vi "Launcher.vi"() -> ()   [LabVIEW 2020]
uses:
  <vilib>/Analysis/6fits.llb/Curve Fitting Criteria.ctl
  <vilib>/Analysis/baseanly.llb/Mean (DBL).vi
  DAQ.lvlibp/D/BingoGithub/DAQ_V000.04/DAQ_Module/DAQ_Base_class/DAQ_Base.lvclass
  DAQ_Base_class/subvi/GlobalData_operation.ctl
  <vilib>/Analysis/NI_AALPro.lvlib
  <vilib>/Analysis/NI_AALBase.lvlib
panel:
  out "模拟量数量":i32
  out "自动采集第1段":dbl[][](graph)
  in  "Tab Control":enum32{"采集模块配置", "采集与调试", "模拟量标定"}(tab)
  in  "DAQSettings":T2={"SampleSettings"={"samples per channel"=100, "SampleRate"=1000.0, "TansMaxLength"=500000.0, "ReadTimeOut"=10.0, "时钟源"=""}, "AI_ChannelSettings"={"AI_SettingsArry"=[]}, "AO_ChannelSettings"={"布尔"=FALSE}, "Cnt_ChannelSettings"={"Cnt_ChannelSettings"=[]}} {"Cnt_ChannelSettings"."Cnt_ChannelSettings"."decoding type" items=["X1"=10090, "X2"=10091, "X4"=10092, "双脉冲计数"=10313]; "Cnt_ChannelSettings"."Cnt_ChannelSettings"."z index phase" items=["A High B High"=10040, "A High B Low"=10041, "A Low B High"=10042, "A Low B Low"=10043, ""=0]; "Cnt_ChannelSettings"."Cnt_ChannelSettings"."单位" items=["Radians"=10273, "Degrees"=10146, "Meters"=10219, "Inches"=10379, "Ticks"=10304, "From Custom Scale"=10065]; "AI_ChannelSettings"."AI_SettingsArry"."标定系数"."Offset" format="%_4g"; "AI_ChannelSettings"."AI_SettingsArry"."标定系数"."Scale" format="%.4g"; "AI_ChannelSettings"."AI_SettingsArry"."shunt resistor location" items=["默认"=-1, "内部"=10200, "外部"=10167]; "AI_ChannelSettings"."AI_SettingsArry"."external shunt resistor value" format="%0.2f"; "AI_ChannelSettings"."AI_SettingsArry"."输入信号类型" items=["默认"=-1, "RSE"=10083, "NRSE"=10078, "差分"=10106, "伪差分"=12529]; "AI_ChannelSettings"."AI_SettingsArry"."单位" items=["安培"=10342, "伏特"=10348, "来自自定义换算"=10065]}
  in  "Save":bool
  in  "ClearCurve":bool
  in  "数据采集通道使能":bool[](array[boolean])
  out "手动采集曲线":dbl[][](graph)
  in  "待标数据源":u16(ring) items=["输入轴扭矩", "输出轴扭矩"]
  in  "tb_sensor_calibrt_data":string[][](table) caption="标定点录入表"
  out "物理值曲线":dbl[](graph)
  in  "Play":bool
  in  "Add":bool
  in  "Remove":bool
  in  "Delete":bool
  in  "Calculate":bool
  in  "Download":bool
  out "real_value":dbl caption="实时值" format="%0.2f"
  out "mean":dbl caption="物理均值" format="%0.2f"
  out "标定拟合曲线":cluster{dbl[], "Best Linear Fit":dbl[]}[](graph)
  out "b_before":dbl caption="计算前偏移量"
  out "K_before":dbl caption="计算前线性度"
  in  "cal_K":dbl caption="计算后线性度"
  in  "cal_b":dbl caption="计算后偏移量"
  out "Stop":bool
  out "自动采集第2段":dbl[][](graph)
  in  "停止":bool
  out "RealTimeValue":dbl[](array[numeric])
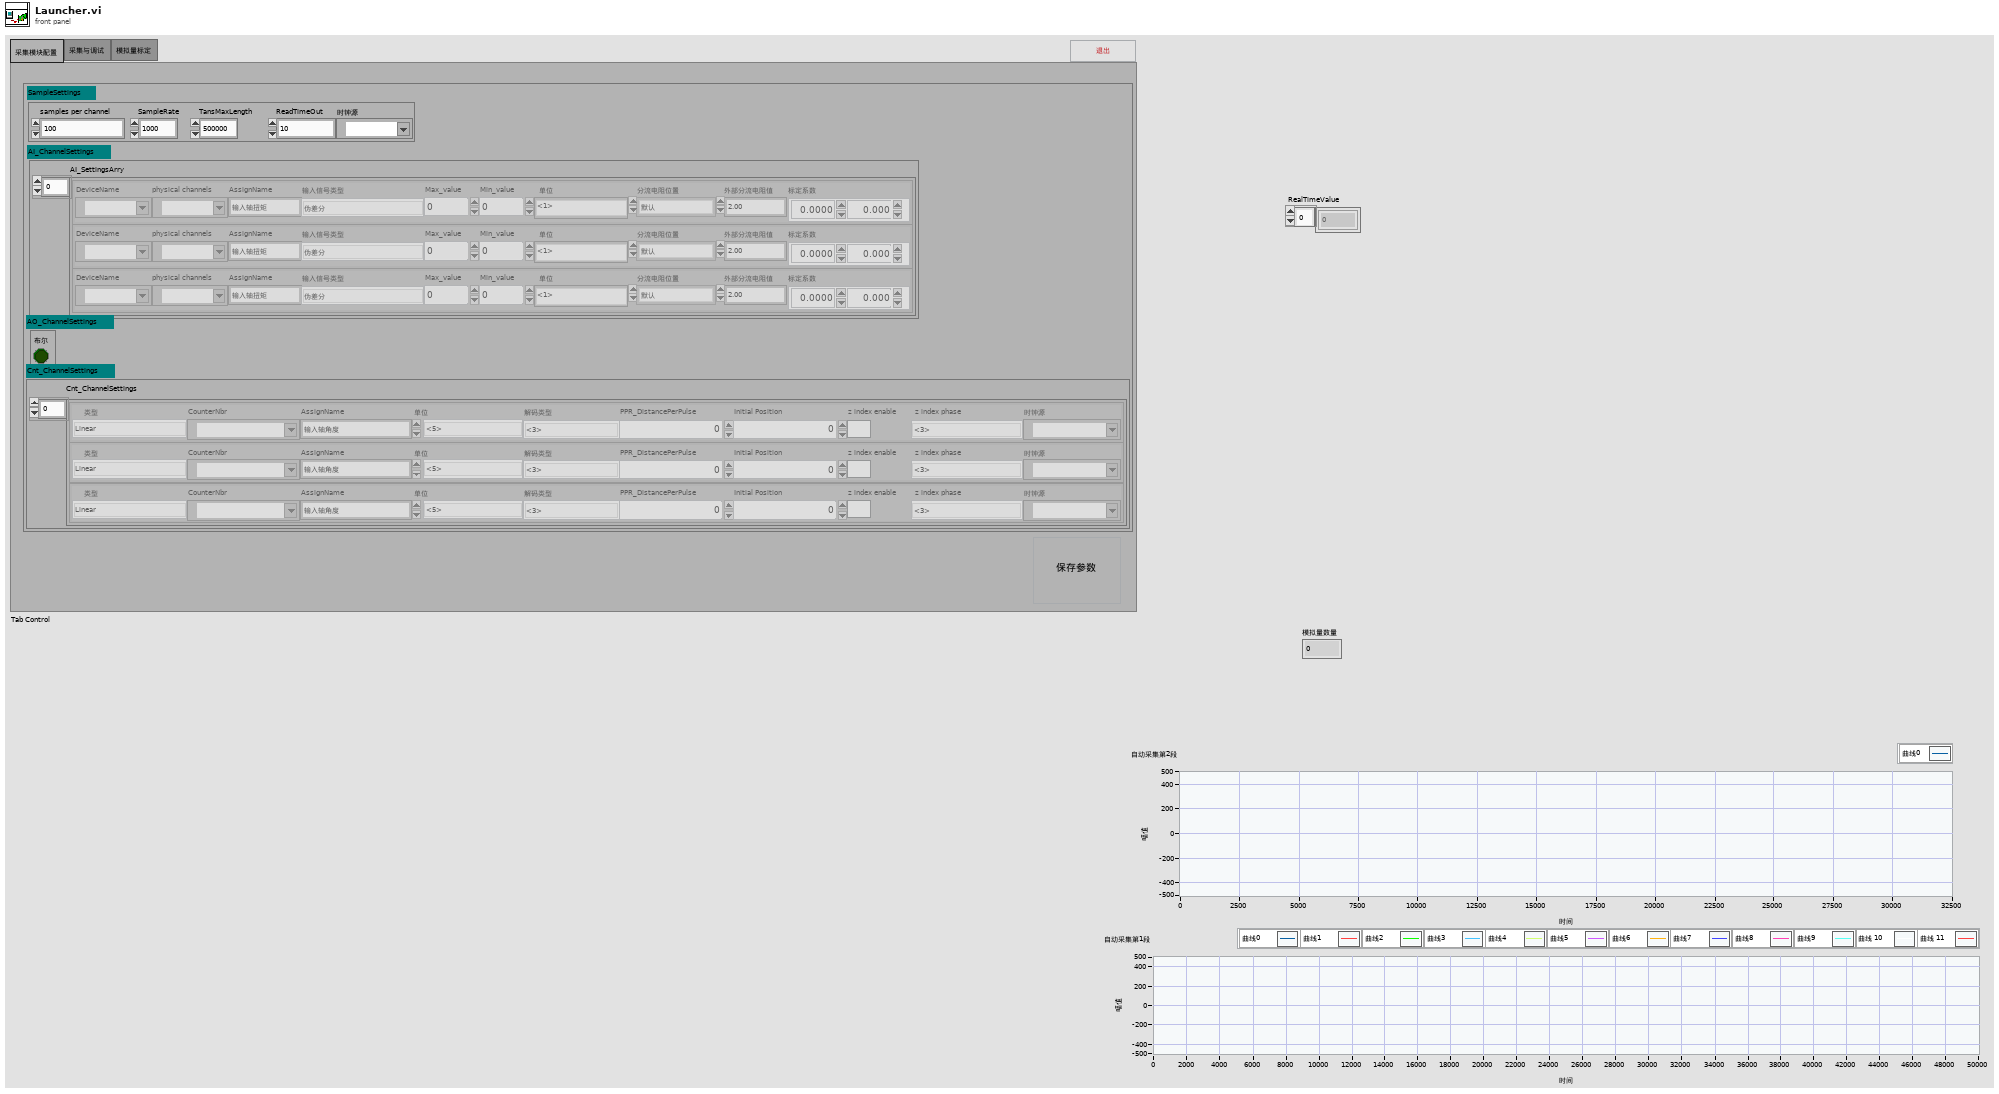
[diagram p1: front panel]
types:
  T1 = typedef "AI信号类型.ctl" = i32
  T2 = cluster{"SampleSettings":cluster{"samples per channel":i32, "SampleRate":dbl, "TansMaxLength":dbl, "ReadTimeOut":dbl, "时钟源":tag}, "AI_ChannelSettings":cluster{"AI_SettingsArry":cluster{"DeviceName":tag, "physical channels":tag, "AssignName":string, "输入信号类型":T1, "Max_value":dbl, "Min_value":dbl, "单位":i32, "shunt resistor location":i32, "external shunt resistor value":dbl, "标定系数":cluster{"Scale":dbl, "Offset":dbl}}[]}, "AO_ChannelSettings":cluster{"布尔":bool}, "Cnt_ChannelSettings":cluster{"Cnt_ChannelSettings":cluster{"类型":enum16{"Linear", "Rotate"}, "CounterNbr":tag, "AssignName":string, "单位":u16, "decoding type":u16, "PPR_DistancePerPulse":dbl, "Initial Position ":dbl, "z index enable":bool, "z index phase":i32, "source":tag}[]}}
  T3 = typedef "DAQ.lvlibp/DAQ_Base.lvclass/DAQSettings.ctl" = cluster{"SampleSettings":T4, "AI_ChannelSettings":T5, "AO_ChannelSettings":T7, "Cnt_ChannelSettings":T8}
  T4 = typedef "DAQ.lvlibp/DAQ_Base.lvclass/SampleSettings.ctl" = cluster{"samples per channel":i32, "SampleRate":dbl, "TansMaxLength":dbl, "ReadTimeOut":dbl, "时钟源":tag}
  T5 = typedef "DAQ.lvlibp/DAQ_Base.lvclass/AI_ChannelSettings.ctl" = cluster{"AI_SettingsArry":cluster{"DeviceName":tag, "physical channels":tag, "AssignName":string, "输入信号类型":T6, "Max_value":dbl, "Min_value":dbl, "单位":i32, "shunt resistor location":i32, "external shunt resistor value":dbl, "标定系数":cluster{"Scale":dbl, "Offset":dbl}}[]}
  T6 = typedef "DAQ.lvlibp/AI信号类型.ctl" = i32
  T7 = typedef "DAQ.lvlibp/DAQ_Base.lvclass/AO_ChannelSettings.ctl" = cluster{"布尔":bool}
  T8 = typedef "DAQ.lvlibp/DAQ_Base.lvclass/Cnt_ChannelSettings.ctl" = cluster{"Cnt_ChannelSettings":cluster{"类型":enum16{"Linear", "Rotate"}, "CounterNbr":tag, "AssignName":string, "单位":u16, "decoding type":u16, "PPR_DistancePerPulse":dbl, "Initial Position ":dbl, "z index enable":bool, "z index phase":i32, "source":tag}[]}
  T9 = typedef "GlobalData_operation.ctl" = enum16{"idle", "read", "write", "clear", "init", "destroy"}
  T10 = typedef "DAQ.lvlibp/DAQ_Base.lvclass/DataCollector.ctl" = cluster{"DataCollectArry":dbl[][], "Update":bool}
  T11 = cluster{"CollectDataQueue":refnum<queue>, "ArryDataCollectorChannel":T10[], "RealTimeValues":dbl[]}
  T12 = typedef "DAQ.lvlibp/DAQ_Base.lvclass/ObjectAttributesRef.ctl" = refnum<data-value>
  T13 = typedef "NI_AALPro.lvlib/Curve Fitting Criteria.ctl" = u16
  T14 = cluster{"DeviceName":tag, "physical channels":tag, "AssignName":string, "输入信号类型":T1, "Max_value":dbl, "Min_value":dbl, "单位":i32, "shunt resistor location":i32, "external shunt resistor value":dbl, "标定系数":cluster{"Scale":dbl, "Offset":dbl}}[]
  T15 = cluster{"DeviceName":tag, "physical channels":tag, "AssignName":string, "输入信号类型":T1, "Max_value":dbl, "Min_value":dbl, "单位":i32, "shunt resistor location":i32, "external shunt resistor value":dbl, "标定系数":cluster{"Scale":dbl, "Offset":dbl}}
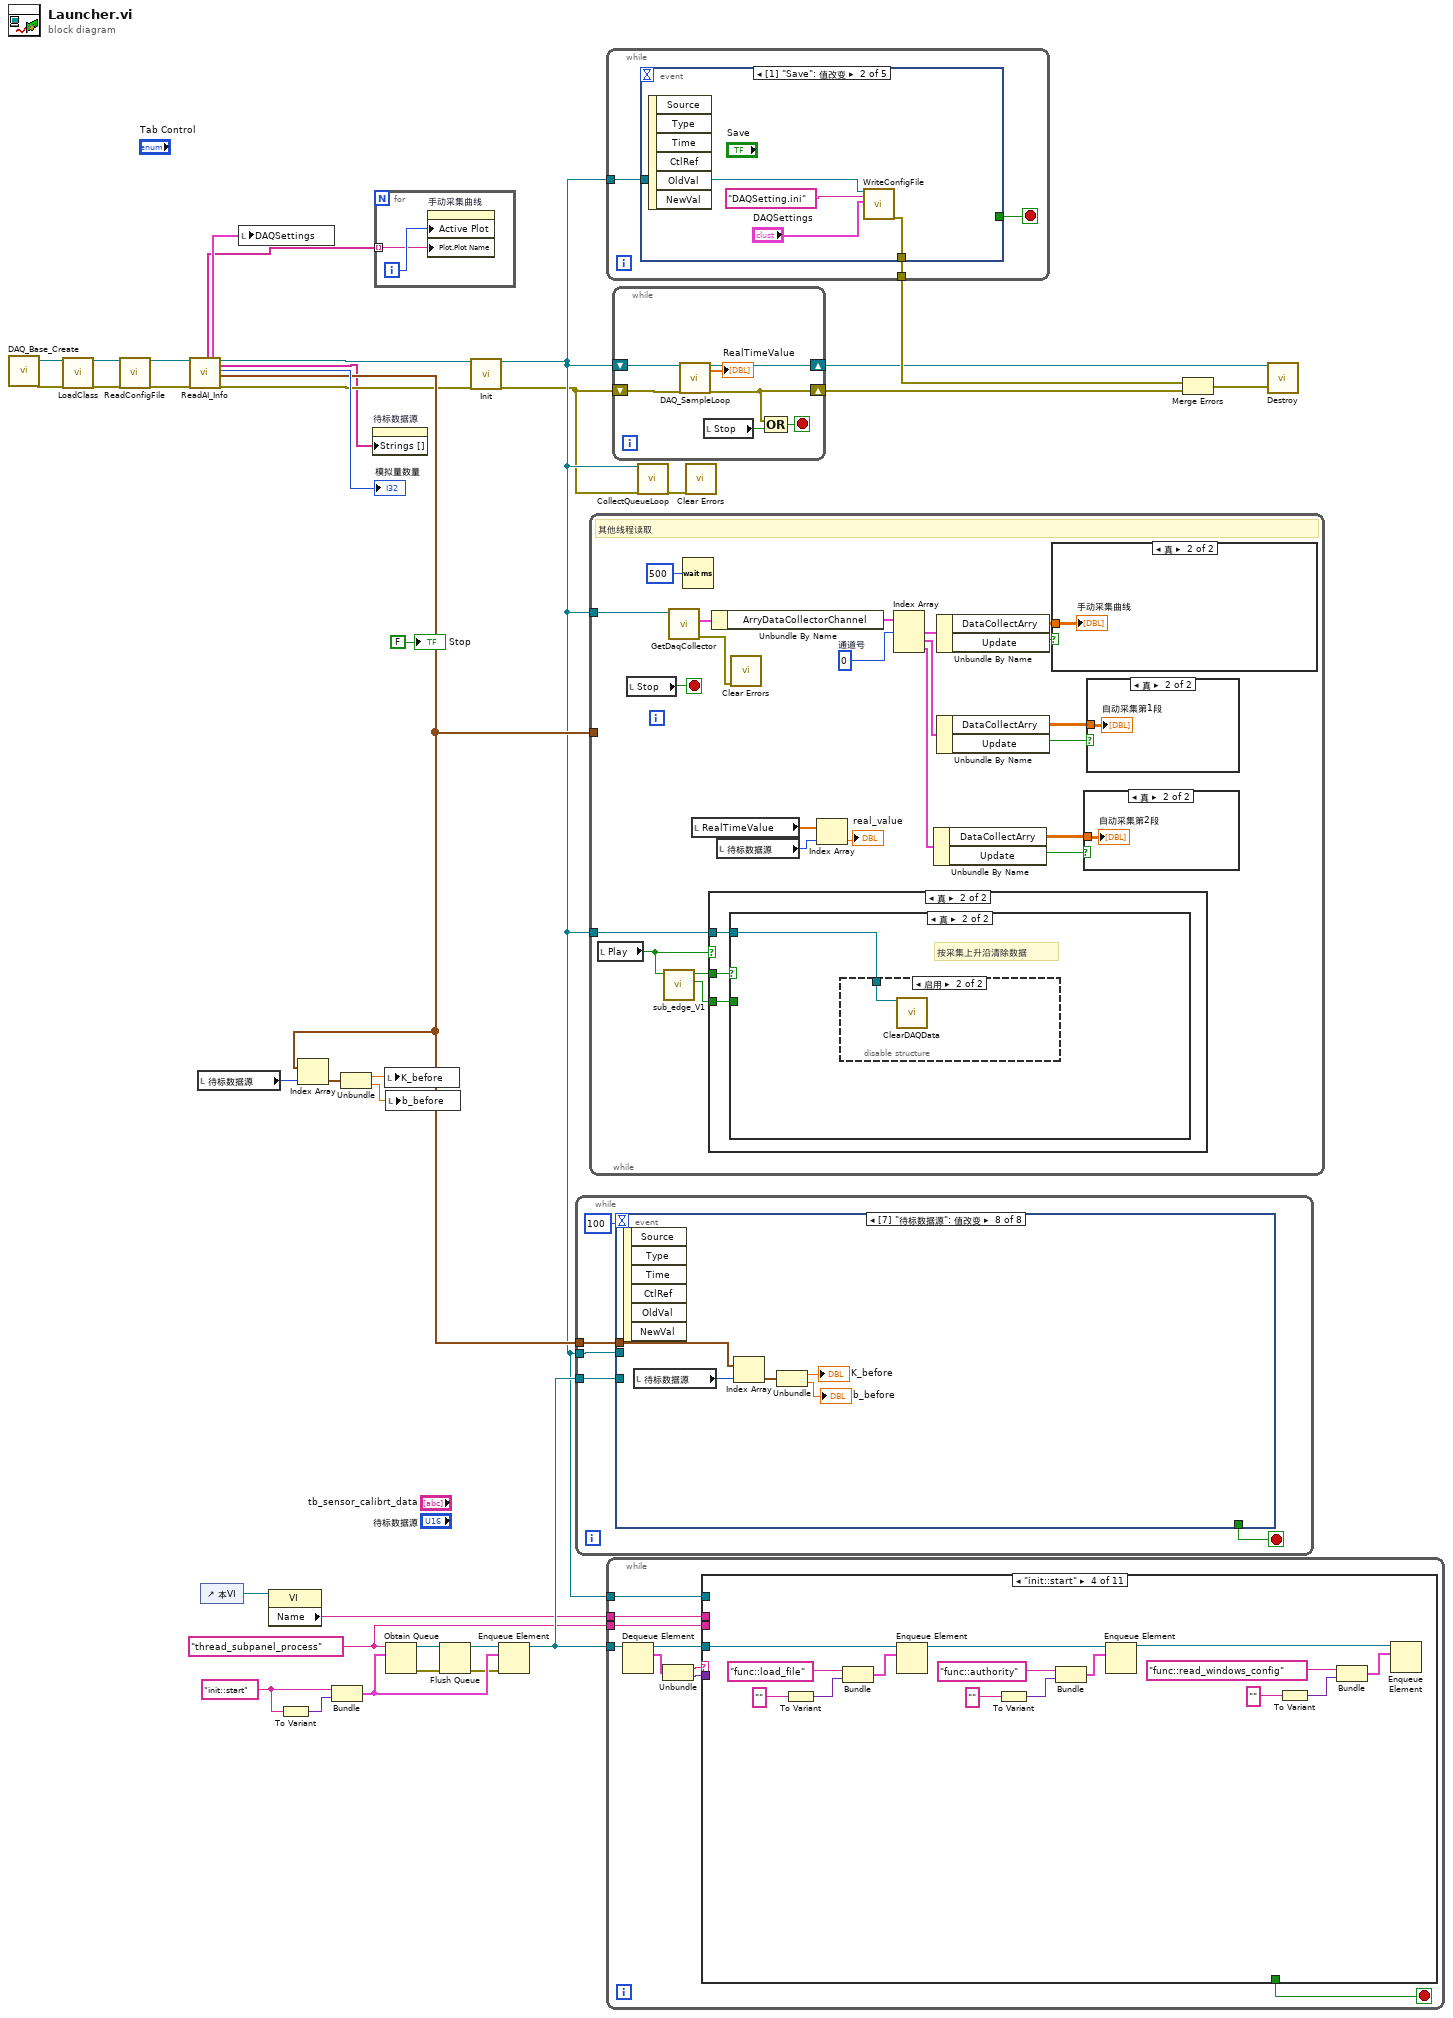
[diagram p0: block diagram]
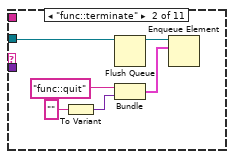
[diagram p3: hidden frame]
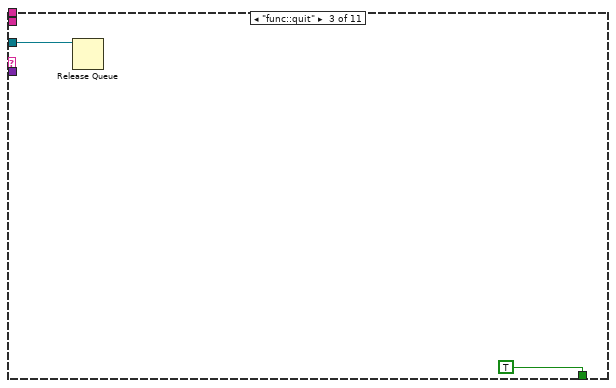
[diagram p4: hidden frame]
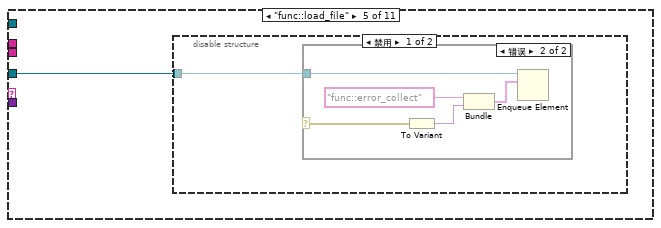
[diagram p5: hidden frame]
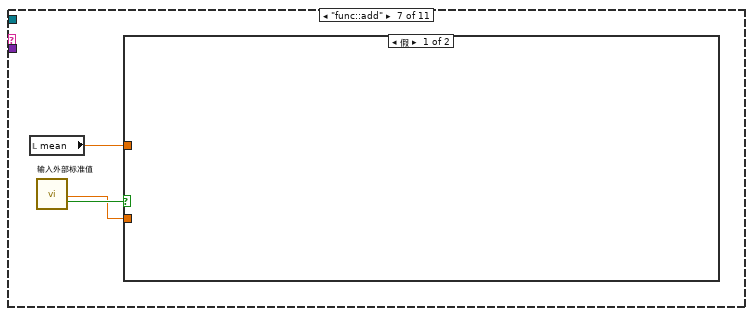
[diagram p9: hidden frame]
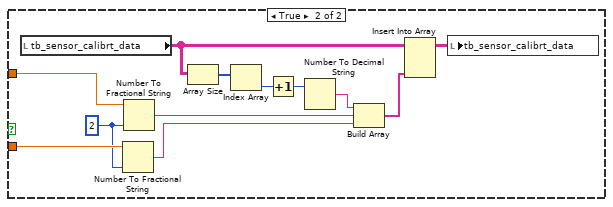
[diagram p10: hidden frame]
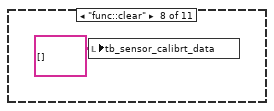
[diagram p11: hidden frame]
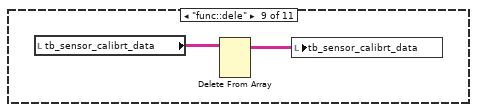
[diagram p12: hidden frame]
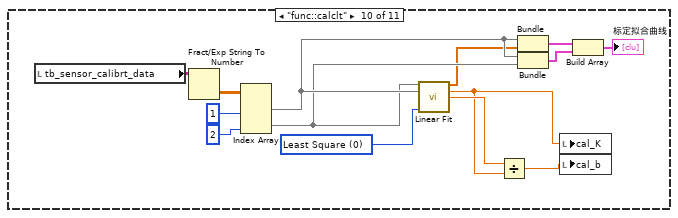
[diagram p13: hidden frame]
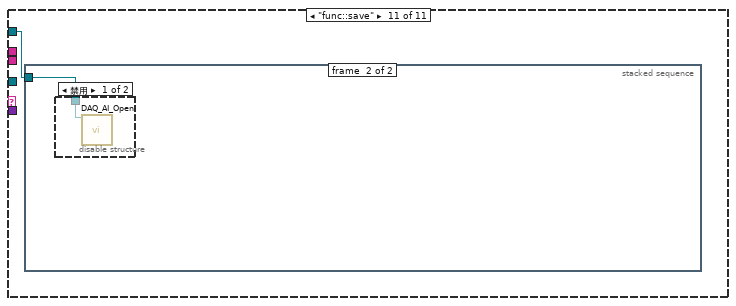
[diagram p14: hidden frame]
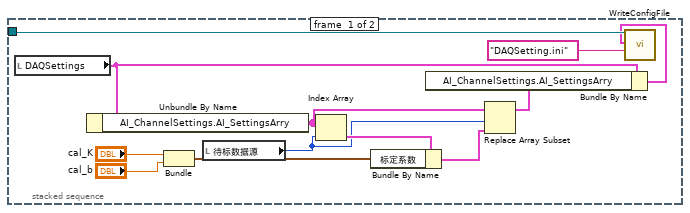
[diagram p15: hidden frame]
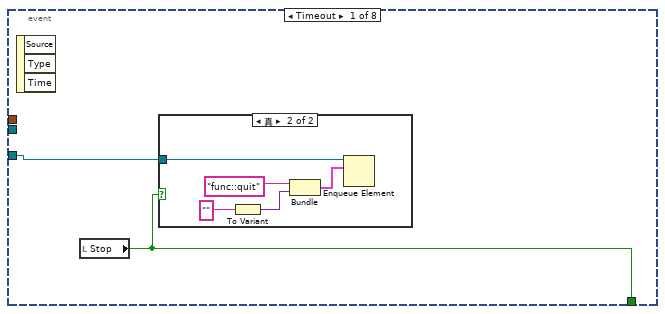
[diagram p17: hidden frame]
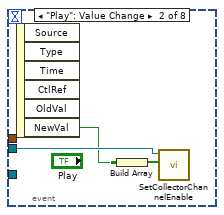
[diagram p19: hidden frame]
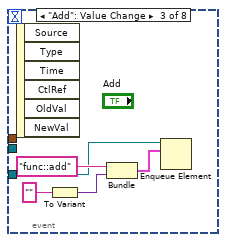
[diagram p20: hidden frame]
diagram:
  w25 = "init::start" ("名称（未命名）")
  w21 = "thread_subpanel_process" ("名称（未命名）")
  n1 = call "DAQ_Base_Create.vi"() -> ("reference out"=w36:refnum<class "DAQ_Base.lvclass">, "error out"=w35:errorcluster)  [unwired: 18 in]
  n2 = call "LoadClass.vi"("reference in"=w36, "error in (no error)"=w35) -> ("reference out"=w5:refnum<class "DAQ_Base.lvclass">, "error out"=w7:errorcluster)  [unwired: 16 in]
  n3 = call-dynamic "ReadConfigFile.vi"("reference in"=w5, "error in (no error)"=w7) -> ("reference out"=w4:refnum<class "DAQ_Base.lvclass">, "error out"=w6:errorcluster)  [unwired: 16 in]
  n4 = call "ReadAI_Info.vi"("reference in"=w4, "error in (no error)"=w6) -> ("采集通道名称"=w1:string[], "DAQSettings"=w3:T3, "reference out"=w11:refnum<class "DAQ_Base.lvclass">, "模拟量名称"=w2:string[], "模拟量数量"=→"模拟量数量":i32, "标定系数Arry"=w17:cluster{"Scale":dbl, "Offset":dbl}[], "error out"=w10:errorcluster)  [unwired: 10 in, 1 out]
  n5 = local read "待标数据源"() -> (w19:u16)
  n6 = control-ref of="本VI"() -> (w24:refnum<vi>)
  n7 = local write "DAQSettings"(w3) -> ()
  n8 = property class="VI"(reference=w24) -> ("Name"=w22:string)  [unwired: 1 in, 2 out]
  n9 = To Variant(anything=w25) -> (Variant=w31:variant)
  n10 = Index Array(array=w17, index=w19) -> (element=w18:cluster{"Scale":dbl, "Offset":dbl})
  n11 = Bundle("名称（未命名）"=w25, "Variant"=w31) -> (w30:cluster{"名称（未命名）":string, "Variant":variant})  [unwired: 1 in]
  n12 = Unbundle(w18) -> ("Scale"=w16:dbl, "Offset"=w15:dbl)
  n13 = property on="待标数据源" class="Ring (严格)"("Strings []"=w2) -> ()  [unwired: 2 in, 2 out]
  n14 = for {
    tunnel: w1 -> [w37] mode=indexing
    i -> [w38]
    n15 = property on="手动采集曲线" class="WFGraph (严格)"("Active Plot"=w38, "Plot.Plot Name"=w37) -> ()  [unwired: 2 in, 2 out]
  }
  n16 = local write "K_before"(w16) -> ()
  n17 = local write "b_before"(w15) -> ()
  n18 = Obtain Queue(name (unnamed)=w21, element data type=w30) -> (queue out=w29:refnum<queue>, error out=w28:errorcluster)  [unwired: 3 in, 1 out]
  n19 = Flush Queue(queue=w29, error in (no error)=w28) -> (queue out=w27:refnum<queue>, error out=w26:errorcluster)  [unwired: 1 out]
  n20 = call-dynamic "Init.vi"("reference in"=w11, "error in (no error)"=w10) -> ("reference out"=w9:refnum<class "DAQ_Base.lvclass">, "error out"=w8:errorcluster)  [unwired: 16 in]
  n21 = Enqueue Element(queue=w27, element=w30, error in (no error)=w26) -> (queue out=w23:refnum<queue>)  [unwired: 1 in, 2 out]
  n22 = while {
    tunnel: w23 -> [w42]
    tunnel: w9 -> [w40]
    tunnel: w17 -> [w39]
    stop <- w43 stop-if-true
    n23 = event shown="[7] \"待标数据源\": 值改变" {
      selector: _ -> [_ _ _ _ _ _ _ _]
      dyn-events: _ -> [_ _ _ _ _ _ _ _]
      timeout: 100 -> [_ _ _ _ _ _ _ _]
      tunnel: [w44 _ _ _ _ _ _ _] -> w43
      tunnel: w42 -> [w45 _ w54 w59 w64 w69 w74 _]
      tunnel: w40 -> [_ w52 _ _ _ _ _ _]
      tunnel: w39 -> [_ _ _ _ _ _ _ w79]
      event Timeout {
        n24 = event-data() -> ()  [unwired: 1 in, 3 out]
        n25 = local read "Stop"() -> (w44:bool)
        n26 = case shown="真" w44 {
          tunnel: w45 -> [_ w46]
          frame False {
          }
          frame True {
            n27 = To Variant(anything="") -> (Variant=w47:variant)
            n28 = Bundle("名称（未命名）"="func::quit", "Variant"=w47) -> (w49:cluster{"名称（未命名）":string, "Variant":variant})  [unwired: 1 in]
            n29 = Enqueue Element(queue=w46, element=w49) -> ()  [unwired: 2 in, 3 out]
          }
        }
      }
      event "Play": Value Change {
        n30 = event-data() -> ("NewVal"=w51:bool)  [unwired: 1 in, 5 out]
        n31 = Build Array(w51) -> (w53:bool[])
        n32 = call-dynamic "SetCollectorChannelEnable.vi"("CollectorChannelEnable"=w53, "reference in"=w52) -> ()  [unwired: 8 in, 2 out]
      }
      event "Add": Value Change {
        n33 = event-data() -> ()  [unwired: 1 in, 6 out]
        n34 = To Variant(anything="") -> (Variant=w58:variant)
        n35 = Bundle("名称（未命名）"="func::add", "Variant"=w58) -> (w56:cluster{"名称（未命名）":string, "Variant":variant})  [unwired: 1 in]
        n36 = Enqueue Element(queue=w54, element=w56) -> ()  [unwired: 2 in, 3 out]
      }
      event "Remove": Value Change {
        n37 = event-data() -> ()  [unwired: 1 in, 6 out]
        n38 = To Variant(anything="") -> (Variant=w63:variant)
        n39 = Bundle("名称（未命名）"="func::dele", "Variant"=w63) -> (w61:cluster{"名称（未命名）":string, "Variant":variant})  [unwired: 1 in]
        n40 = Enqueue Element(queue=w59, element=w61) -> ()  [unwired: 2 in, 3 out]
      }
      event "Delete": Value Change {
        n41 = event-data() -> ()  [unwired: 1 in, 6 out]
        n42 = To Variant(anything="") -> (Variant=w68:variant)
        n43 = Bundle("名称（未命名）"="func::clear", "Variant"=w68) -> (w66:cluster{"名称（未命名）":string, "Variant":variant})  [unwired: 1 in]
        n44 = Enqueue Element(queue=w64, element=w66) -> ()  [unwired: 2 in, 3 out]
      }
      event "Calculate": Value Change {
        n45 = event-data() -> ()  [unwired: 1 in, 6 out]
        n46 = To Variant(anything="") -> (Variant=w73:variant)
        n47 = Bundle("名称（未命名）"="func::calclt", "Variant"=w73) -> (w71:cluster{"名称（未命名）":string, "Variant":variant})  [unwired: 1 in]
        n48 = Enqueue Element(queue=w69, element=w71) -> ()  [unwired: 2 in, 3 out]
      }
      event "Download": Value Change {
        n49 = event-data() -> ()  [unwired: 1 in, 6 out]
        n50 = To Variant(anything="") -> (Variant=w78:variant)
        n51 = Bundle("名称（未命名）"="func::save", "Variant"=w78) -> (w76:cluster{"名称（未命名）":string, "Variant":variant})  [unwired: 1 in]
        n52 = Enqueue Element(queue=w74, element=w76) -> ()  [unwired: 2 in, 3 out]
      }
      event "待标数据源": Value Change {
        n53 = event-data() -> ()  [unwired: 1 in, 6 out]
        n54 = local read "待标数据源"() -> (w80:u16)
        n55 = Index Array(array=w79, index=w80) -> (element=w81:cluster{"Scale":dbl, "Offset":dbl})
        n56 = Unbundle(w81) -> ("Scale"=→"K_before":dbl, "Offset"=→"b_before":dbl)
      }
    }
  }
  n57 = while {
    tunnel: w9 -> [w105]
    tunnel: w9 -> [w87]
    tunnel: w17 -> [_]
    stop <- w91 stop-if-true
    w99 = 0  # 通道号
    # "其他线程读取"
    n58 = local read "Play"() -> (w90:bool)
    n59 = local read "Stop"() -> (w91:bool)
    n60 = call "sub_edge_V1.vi"("signal_in"=w90) -> ("fail_edge"=w89:bool, "raise_edge"=w88:bool)  [unwired: 8 in, 1 out]
    n61 = call-dynamic "GetDaqCollector.vi"("reference in"=w105) -> ("error out"=w92:errorcluster, "DaqCollector"=w104:T11)  [unwired: 8 in, 1 out]
    n62 = Wait (ms)(milliseconds to wait=u32 500 ("等待时间（毫秒）")) -> ()  [unwired: 1 out]
    n63 = local read "RealTimeValue"() -> (w84:dbl[])
    n64 = case shown="真" w90 {
      tunnel: w88 -> [_ w120]
      tunnel: w89 -> [w107 w119]
      tunnel: w87 -> [_ w118]
      frame False {
        n65 = case shown="假" w107 {
          frame False {
          }
          frame True {
            # "采集按钮下降沿计算一下均值"
            n66 = local read "手动采集曲线"() -> (w111:dbl[][])
            n67 = local read "模拟量数量"() -> (w112:i32)
            n68 = Array Size(array=w111) -> (size(s)=w114:i32[])
            n69 = Index Array(array=w114) -> (element #1=w113:i32)  [unwired: 2 in, 1 out]
            n70 = Subtract(x=w113, y=w112) -> (x-y=w110:i32)
            n71 = local read "待标数据源"() -> (w115:u16)
            n72 = Delete From Array(array=w111, length=3 ("长度"), index (row)=w110) -> (deleted portion=w108:dbl[][])  [unwired: 1 in, 1 out]
            n73 = Index Array(array=w108, index (row)=w115) -> (element=w117:dbl[])  [unwired: 1 in]
            n74 = call-poly <vilib>:"Mean.vi"("X"=w117) -> ("mean"=→"mean":dbl)  [unwired: 1 out]
          }
        }
      }
      frame True {
        n75 = case shown="真" w120 {
          tunnel: w119 -> [w121 _]
          tunnel: w118 -> [_ w131]
          frame False {
            n76 = case shown="真" w121 {
              frame False {
                # "显示物理值曲线"
                n77 = local read "手动采集曲线"() -> (w126:dbl[][])
                n78 = local read "模拟量数量"() -> (w127:i32)
                n79 = Array Size(array=w126) -> (size(s)=w129:i32[])
                n80 = Index Array(array=w129) -> (element #1=w128:i32)  [unwired: 2 in, 1 out]
                n81 = local read "待标数据源"() -> (w130:u16)
                n82 = Subtract(x=w128, y=w127) -> (x-y=w125:i32)
                n83 = Delete From Array(array=w126, length=3 ("长度"), index (row)=w125) -> (deleted portion=w124:dbl[][])  [unwired: 1 in, 1 out]
                n84 = Index Array(array=w124, index (row)=w130) -> (element=→"物理值曲线":dbl[])  [unwired: 1 in]
              }
              frame True {
              }
            }
          }
          frame True {
            # "按采集上升沿清除数据"
            n85 = disable-structure shown="启用" {
              disable-tunnel: w131 -> [w132 w136]
              frame Disabled {
                n86 = call "DAQ_Base_GetAttributes.vi"("reference in"=w132, "return data? (T)"=FALSE) -> ("attributes ref"=w134:T12)  [unwired: 14 in, 3 out]
                n87 = call "GlobalCollectDataRefOperate.vi"("operation"=GlobalData_operation."clear", "attributes ref"=w134) -> ()  [unwired: 7 in, 3 out]
              }
              frame Enabled {
                n88 = call "ClearDAQData.vi"("reference in"=w136) -> ()  [unwired: 17 in, 2 out]
              }
            }
          }
        }
      }
    }
    n89 = Unbundle By Name(w104) -> ("ArryDataCollectorChannel"=w103:T10[])
    n90 = local read "待标数据源"() -> (w85:u16)
    n91 = call <vilib>:"Clear Errors.vi"("error in (no error)"=w92) -> ()  [unwired: 5 in, 2 out]
    n92 = Index Array(array=w84, index=w85) -> (element=→"real_value":dbl)
    n93 = Index Array(array=w103, index #1=w99) -> (element #1=w102:T10, element #2=w94:T10, element #3=w93:T10)  [unwired: 2 in]
    n94 = Unbundle By Name(w93) -> ("DataCollectArry"=w95:dbl[][], "Update"=w96:bool)
    n95 = Unbundle By Name(w102) -> ("DataCollectArry"=w100:dbl[][], "Update"=w101:bool)
    n96 = Unbundle By Name(w94) -> ("DataCollectArry"=w98:dbl[][], "Update"=w97:bool)
    n97 = case shown="真" w101 {
      tunnel: w100 -> [_ w139]
      frame False {
      }
      frame True {
        "手动采集曲线" <- w139
      }
    }
    n98 = case shown="真" w96 {
      tunnel: w95 -> [_ w137]
      frame False {
      }
      frame True {
        "自动采集第2段" <- w137
      }
    }
    n99 = case shown="真" w97 {
      tunnel: w98 -> [_ w138]
      frame False {
      }
      frame True {
        "自动采集第1段" <- w138
      }
    }
  }
  n100 = while {
    tunnel: w9 -> [w142]
    tunnel: [w140] -> w13
    stop <- w141 stop-if-true
    n101 = event shown="[1] \"Save\": 值改变" {
      selector: _ -> [_ _ _ _ _]
      dyn-events: _ -> [_ _ _ _ _]
      timeout: _ -> [_ _ _ _ _]
      tunnel: w142 -> [_ w145 _ w148 w154]
      tunnel: [_ _ w147 _ _] -> w141
      tunnel: [_ w143 _ _ _] -> w140
      event Timeout {
        n102 = event-data() -> ()  [unwired: 1 in, 3 out]
      }
      event "Save": Value Change {
        n103 = event-data() -> ()  [unwired: 1 in, 6 out]
        n104 = call-dynamic "WriteConfigFile.vi"("reference in"=w145, "ConfigFlieName"="DAQSetting.ini", "DAQSettings"="DAQSettings") -> ("error out"=w143:errorcluster)  [unwired: 15 in, 1 out]
      }
      event "停止": Value Change {
        n105 = event-data() -> ("NewVal"=w147:bool)  [unwired: 1 in, 5 out]
        n106 = local write "Stop"(w147) -> ()
      }
      event "ClearCurve": Value Change {
        n107 = event-data() -> ()  [unwired: 1 in, 6 out]
        n108 = disable-structure shown="启用" {
          disable-tunnel: w148 -> [w149 w153]
          frame Disabled {
            n109 = call "DAQ_Base_GetAttributes.vi"("reference in"=w149, "return data? (T)"=FALSE) -> ("attributes ref"=w151:T12)  [unwired: 14 in, 3 out]
            n110 = call "GlobalCollectDataRefOperate.vi"("operation"=GlobalData_operation."clear", "attributes ref"=w151) -> ()  [unwired: 7 in, 3 out]
          }
          frame Enabled {
            n111 = call "ClearDAQData.vi"("reference in"=w153) -> ()  [unwired: 17 in, 2 out]
          }
        }
      }
      event "数据采集通道使能": Value Change {
        n112 = event-data() -> ()  [unwired: 1 in, 6 out]
        n113 = call-dynamic "SetCollectorChannelEnable.vi"("CollectorChannelEnable"="数据采集通道使能", "reference in"=w154) -> ()  [unwired: 8 in, 2 out]
      }
    }
  }
  n114 = while {
    tunnel: w23 -> [w164]
    tunnel: w22 -> [w159]
    tunnel: w21 -> [w158]
    tunnel: w9 -> [w156]
    stop <- w160 stop-if-true
    n115 = Dequeue Element(queue=w164) -> (queue out=w161:refnum<queue>, element=w163:cluster{"名称（未命名）":string, "Variant":variant})  [unwired: 2 in, 2 out]
    n116 = Unbundle(w163) -> ("名称（未命名）"=w162:string, "Variant"=w157:variant)
    n117 = case shown="\"init::start\"" w162 {
      tunnel: w161 -> [_ w165 w172 w178 w188 _ _ _ _ _ _]
      tunnel: [_ _ TRUE _ _ _ _ _ _ _ _] -> w160
      tunnel: w159 -> [_ _ _ _ _ _ _ _ _ _ _]
      tunnel: w158 -> [_ _ _ _ _ _ _ _ _ _ _]
      tunnel: w157 -> [_ _ _ _ _ _ _ _ _ _ _]
      tunnel: w156 -> [_ _ _ _ _ _ _ _ _ _ w227]
      frame "假", Default {
      }
      frame "func::terminate" {
        n118 = To Variant(anything="" ("名称（未命名）")) -> (Variant=w167:variant)
        n119 = Flush Queue(queue=w165) -> (queue out=w166:refnum<queue>)  [unwired: 1 in, 2 out]
        n120 = Bundle("名称（未命名）"="func::quit", "Variant"=w167) -> (w170:cluster{"名称（未命名）":string, "Variant":variant})  [unwired: 1 in]
        n121 = Enqueue Element(queue=w166, element=w170) -> ()  [unwired: 2 in, 3 out]
      }
      frame "func::quit" {
        n122 = Release Queue(queue=w172) -> ()  [unwired: 2 in, 3 out]
      }
      frame "init::start" {
        n123 = To Variant(anything="") -> (Variant=w187:variant)
        n124 = Bundle("名称（未命名）"="func::load_file", "Variant"=w187) -> (w185:cluster{"名称（未命名）":string, "Variant":variant})  [unwired: 1 in]
        n125 = Enqueue Element(queue=w178, element=w185) -> (queue out=w179:refnum<queue>)  [unwired: 2 in, 2 out]
        n126 = To Variant(anything="") -> (Variant=w183:variant)
        n127 = Bundle("名称（未命名）"="func::authority", "Variant"=w183) -> (w181:cluster{"名称（未命名）":string, "Variant":variant})  [unwired: 1 in]
        n128 = Enqueue Element(queue=w179, element=w181) -> (queue out=w173:refnum<queue>)  [unwired: 2 in, 2 out]
        n129 = To Variant(anything="") -> (Variant=w174:variant)
        n130 = Bundle("名称（未命名）"="func::read_windows_config", "Variant"=w174) -> (w176:cluster{"名称（未命名）":string, "Variant":variant})  [unwired: 1 in]
        n131 = Enqueue Element(queue=w173, element=w176) -> ()  [unwired: 2 in, 3 out]
      }
      frame "func::load_file" {
        n132 = disable-structure shown="禁用" {
          disable-tunnel: w188 -> [w189 _]
          frame Disabled {
            n133 = case shown="错误" {
              selector: _ -> [_ w190]
              tunnel: w189 -> [_ w191]
              frame No Error {
              }
              frame Error {
                n134 = To Variant(anything=w190) -> (Variant=w194:variant)
                n135 = Bundle("名称（未命名）"="func::error_collect", "Variant"=w194) -> (w192:cluster{"名称（未命名）":string, "Variant":variant})  [unwired: 1 in]
                n136 = Enqueue Element(queue=w191, element=w192) -> ()  [unwired: 2 in, 3 out]
              }
            }
          }
          frame Enabled {
          }
        }
      }
      frame "func::authority" {
      }
      frame "func::add" {
        n137 = local read "mean"() -> (w195:dbl)
        n138 = call "输入外部标准值"() -> ("外部标准值"=w196:dbl, "OK"=w197:bool)  [unwired: 17 in, 1 out]
        n139 = case shown="假" w197 {
          tunnel: w195 -> [_ w205]
          tunnel: w196 -> [_ w204]
          frame False {
          }
          frame True {
            w203 = i16 2 ("precision (6)")
            n140 = local read "tb_sensor_calibrt_data"() -> (w209:string[][])
            n141 = Number To Fractional String(number=w204, precision (6)=w203) -> (F-format string=w199:string)  [unwired: 2 in]
            n142 = Number To Fractional String(number=w205, precision (6)=w203) -> (F-format string=w200:string)  [unwired: 2 in]
            n143 = Array Size(array=w209) -> (size(s)=w208:i32[])
            n144 = Index Array(array=w208) -> (element=w206:i32)  [unwired: 1 in]
            n145 = Increment(x=w206) -> (x+1=w202:i32)
            n146 = Number To Decimal String(number=w202) -> (decimal integer string=w201:string)  [unwired: 1 in]
            n147 = Build Array(w201, w200, w199) -> (w198:string[])
            n148 = Insert Into Array(array=w209, new element=w198) -> (w207:string[][])  [unwired: 2 in]
            n149 = local write "tb_sensor_calibrt_data"(w207) -> ()
          }
        }
      }
      frame "func::clear" {
        n150 = local write "tb_sensor_calibrt_data"(string[][] [] ("tb_LEM_calibrt_data")) -> ()
      }
      frame "func::dele" {
        n151 = local read "tb_sensor_calibrt_data"() -> (w212:string[][])
        n152 = Delete From Array(array=w212) -> (array with subset deleted=w211:string[][])  [unwired: 3 in, 1 out]
        n153 = local write "tb_sensor_calibrt_data"(w211) -> ()
      }
      frame "func::calclt" {
        w222 = T13 0 items=["Least Square", "Least Absolute Residual", "Bisquare"] ("method")
        n154 = local read "tb_sensor_calibrt_data"() -> (w224:string[][])
        n155 = Fract/Exp String To Number(string=w224) -> (number=w223:dbl[][])  [unwired: 3 in, 1 out]
        n156 = Index Array(array=w223, index (col) #1=1 ("disabled index (col)"), index (col) #2=2 ("disabled index (col)")) -> (element #1=w221:dbl[], element #2=w216:dbl[])  [unwired: 2 in]
        n157 = call <vilib>:"Linear Fit.vi"("Y"=w216, "X"=w221, "method"=w222) -> ("Best Linear Fit"=w215:dbl[], "slope"=w214:dbl, "intercept"=w217:dbl)  [unwired: 8 in, 2 out]
        n158 = Divide(x=w217, y=w214) -> (x/y=w213:dbl)
        n159 = Bundle(w221, "Best Linear Fit"=w215) -> (w220:cluster{dbl[], "Best Linear Fit":dbl[]})  [unwired: 1 in]
        n160 = Bundle(w221, w216) -> (w219:cluster{dbl[], dbl[]})  [unwired: 1 in]
        n161 = local write "cal_K"(w214) -> ()
        n162 = local write "cal_b"(w213) -> ()
        n163 = Build Array(w220, w219) -> (→"标定拟合曲线":cluster{dbl[], "Best Linear Fit":dbl[]}[])
      }
      frame "func::save" {
        n164 = stacked-sequence {
          tunnel: w227 -> [w239 w240]
          frame #0 {
            n165 = local read "DAQSettings"() -> (w229:T2)
            n166 = Unbundle By Name(w229) -> ("AI_ChannelSettings.AI_SettingsArry"=w234:T14)
            n167 = Bundle("cal_K"="cal_K", "cal_b"="cal_b") -> (w235:cluster{"cal_K":dbl, "cal_b":dbl})  [unwired: 1 in]
            n168 = local read "待标数据源"() -> (w233:u16)
            n169 = Index Array(array=w234, index=w233) -> (element=w236:T15)
            n170 = Bundle By Name(cluster=w236, "标定系数"=w235) -> (w232:T15)
            n171 = Replace Array Subset(array=w234, new element=w232, index=w233) -> (w231:T14)
            n172 = Bundle By Name(cluster=w229, "AI_ChannelSettings.AI_SettingsArry"=w231) -> (w228:T2)
            n173 = call-dynamic "WriteConfigFile.vi"("reference in"=w239, "ConfigFlieName"="DAQSetting.ini", "DAQSettings"=w228) -> ()  [unwired: 15 in, 2 out]
          }
          frame #1 {
            n174 = disable-structure shown="禁用" {
              disable-tunnel: w240 -> [w241 _]
              frame Disabled {
                n175 = call-dynamic "DAQ_AI_Open.vi"("reference in"=w241) -> ()  [unwired: 17 in, 2 out]
              }
              frame Enabled {
              }
            }
          }
        }
      }
    }
  }
  n176 = while {
    shift-right: [w248] -> w12
    shift-left: w9 -> [w247]
    shift-right: [w244] -> w34
    shift-left: w8 -> [w246]
    stop <- w245 stop-if-true
    n177 = call-dynamic "DAQ_SampleLoop.vi"("reference in"=w247, "error in (no error)"=w246) -> ("reference out"=w248:refnum<class "DAQ_Base.lvclass">, "RealTimeValue"=→"RealTimeValue":dbl[], "error out"=w244:errorcluster)  [unwired: 15 in]
    n178 = local read "Stop"() -> (w242:bool)
    n179 = Compound Arithmetic op=OR ("复合运算")(w244, w242) -> (w245:bool)
  }
  n180 = call-dynamic "CollectQueueLoop.vi"("reference in"=w9, "error in (no error)"=w8) -> ("error out"=w33:errorcluster)  [unwired: 16 in, 1 out]
  n181 = call <vilib>:"Clear Errors.vi"("error in (no error)"=w33) -> ()  [unwired: 5 in, 2 out]
  n182 = Merge Errors(w13, w34) -> (w14:errorcluster)
  n183 = call-dynamic "Destroy.vi"("reference in"=w12, "error in (no error)"=w14) -> ()  [unwired: 16 in, 2 out]
  "Stop" <- FALSE ("Stop")
